vi "Get Plugin Subset.vi"(10 "plugin index":i32, 11 "plugin group counts":u8[](array[numeric])) -> (2 "length":u8, 3 "index":i32)   [LabVIEW 2017, in "DSF Core.lvlib" / "Framework Status.lvclass"]
uses:
  Framework Status.lvclass
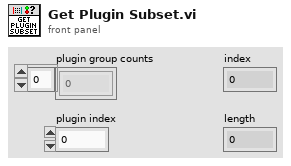
[diagram p1: front panel]
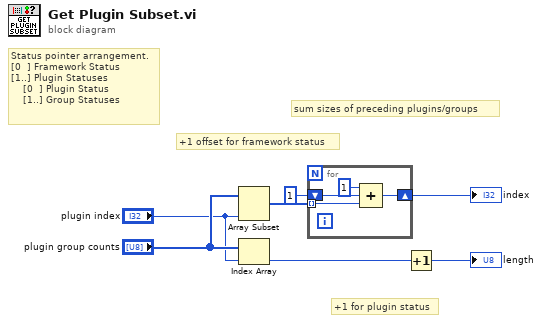
[diagram p0: block diagram]
diagram:
  # "Status pointer arrangement.\n[0  ] Framework Status\n[1..] Plugin Statuses\n    [0  ] Plugin Status\n    [1..] Group Statuses"
  # "sum sizes of preceding plugins/groups"
  # "+1 for plugin status"
  # "+1 offset for framework status"
  n1 = Array Subset(array="plugin group counts", length="plugin index") -> (w2:u8[])  [unwired: 1 in]
  n2 = Index Array(array="plugin group counts", index="plugin index") -> (element=w5:u8)
  n3 = for {
    tunnel: w2 -> [w11] mode=indexing
    shift-right: [w9] -> w6
    shift-left: 1 ("Numeric") -> [w10]
    n4 = Compound Arithmetic op=ADD(1 ("value"), w10, w11) -> (w9:i32)
  }
  "index" <- w6
  n5 = Increment(x=w5) -> (x+1=→"length":u8)
